vi "CreateNew_Invoke.vi"(10 "Cluster":T1, 11 "Wizard":T2) -> (3 "Canceled":bool)   [LabVIEW 2020, in "FlexWorker_Provider.lvlib"]
uses:
  FlexWorker_Provider.lvlib
  <resource>/Framework/Providers/API/ItemRef.ctl
  <resource>/Framework/Providers/API/mxLvNIIM.ctl
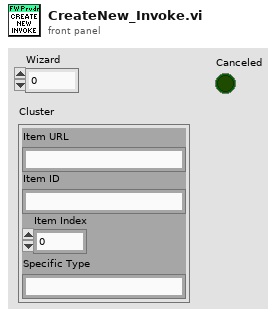
[diagram p1: front panel]
types:
  T1 = typedef "mxLvNIIM.ctl" = cluster{"Item URL":string, "Item ID":string, "Item Index":i32, "Specific Type":string}
  T2 = typedef "ItemRef.ctl" = u64
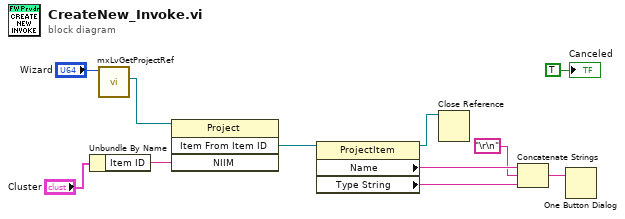
[diagram p0: block diagram]
diagram:
  n1 = Unbundle By Name("Cluster") -> ("Item ID"=w8:string)
  n2 = call <resource>:"mxLvGetProjectRef.vi"("Item"="Wizard") -> ("Project Refnum"=w10:refnum<vi>)  [unwired: 8 in, 2 out]
  n3 = invoke class="Project" method="Item From Item ID"(reference=w10, "NIIM"=w8) -> ("GetItemFromNIIM"=w7:refnum<vi>)  [unwired: 2 in, 3 out]
  n4 = property class="ProjectItem"(reference=w7) -> (reference out=w1:refnum<vi>, "Name"=w6:string, "Type String"=w5:string)  [unwired: 1 in, 1 out]
  n5 = Close Reference(reference=w1) -> ()  [unwired: 1 in, 1 out]
  n6 = Concatenate Strings(w6, "\r\n", w5) -> (w3:string)
  n7 = One Button Dialog(message=w3) -> ()  [unwired: 1 in, 1 out]
  "Canceled" <- TRUE ("Canceled")
